vi "copy and overlay delete.vi"(2 "error in (no error)":errorcluster, 3 "Image Dst":T1, 4 "Image in":T1) -> (0 "error out":errorcluster, 1 "Image Out":T1)   [LabVIEW 2013]
uses:
  <vilib>/vision/Image Controls.llb/IMAQ Image.ctl
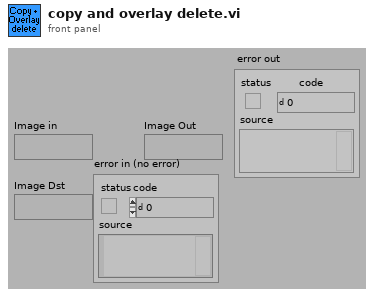
[diagram p1: front panel]
types:
  T1 = typedef "IMAQ Image.ctl" = refnum<image>
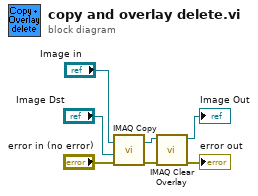
[diagram p0: block diagram]
diagram:
  n1 = call "IMAQ Copy"("error in (no error)"="error in (no error)", "Image Dst"="Image Dst", "Image Src"="Image in") -> ("error out"=w2:errorcluster, "Image Dst Out"=w6:T1)  [unwired: 3 in]
  n2 = call "IMAQ Clear Overlay"("error in (no error)"=w2, "Image"=w6) -> ("error out"=→"error out":errorcluster, "Image Out"=→"Image Out":T1)  [unwired: 8 in]
